vi "Test Get VIs.vi"(8 "Error In":errorcluster) -> ()   [LabVIEW 2018]
uses:
  <vilib>/Utility/traverseref.llb/TRef TravTarget.ctl
  <vilib>/Utility/traverseref.llb/VI Scripting - Traverse.lvlib
panel:
  out "Wires and connected ClassNames in for loop.":string[][](array[string])
  out "Objects[] in for loop":string[](array[string])
  out "All Objects[]":string[](array[string])
  in  "vi path":path=path "C:/Users/lubo/Documents/LabView/LabVIEW-Universal-Transcriptor/Test/Examples For Parsing/Example Test 1.vi"
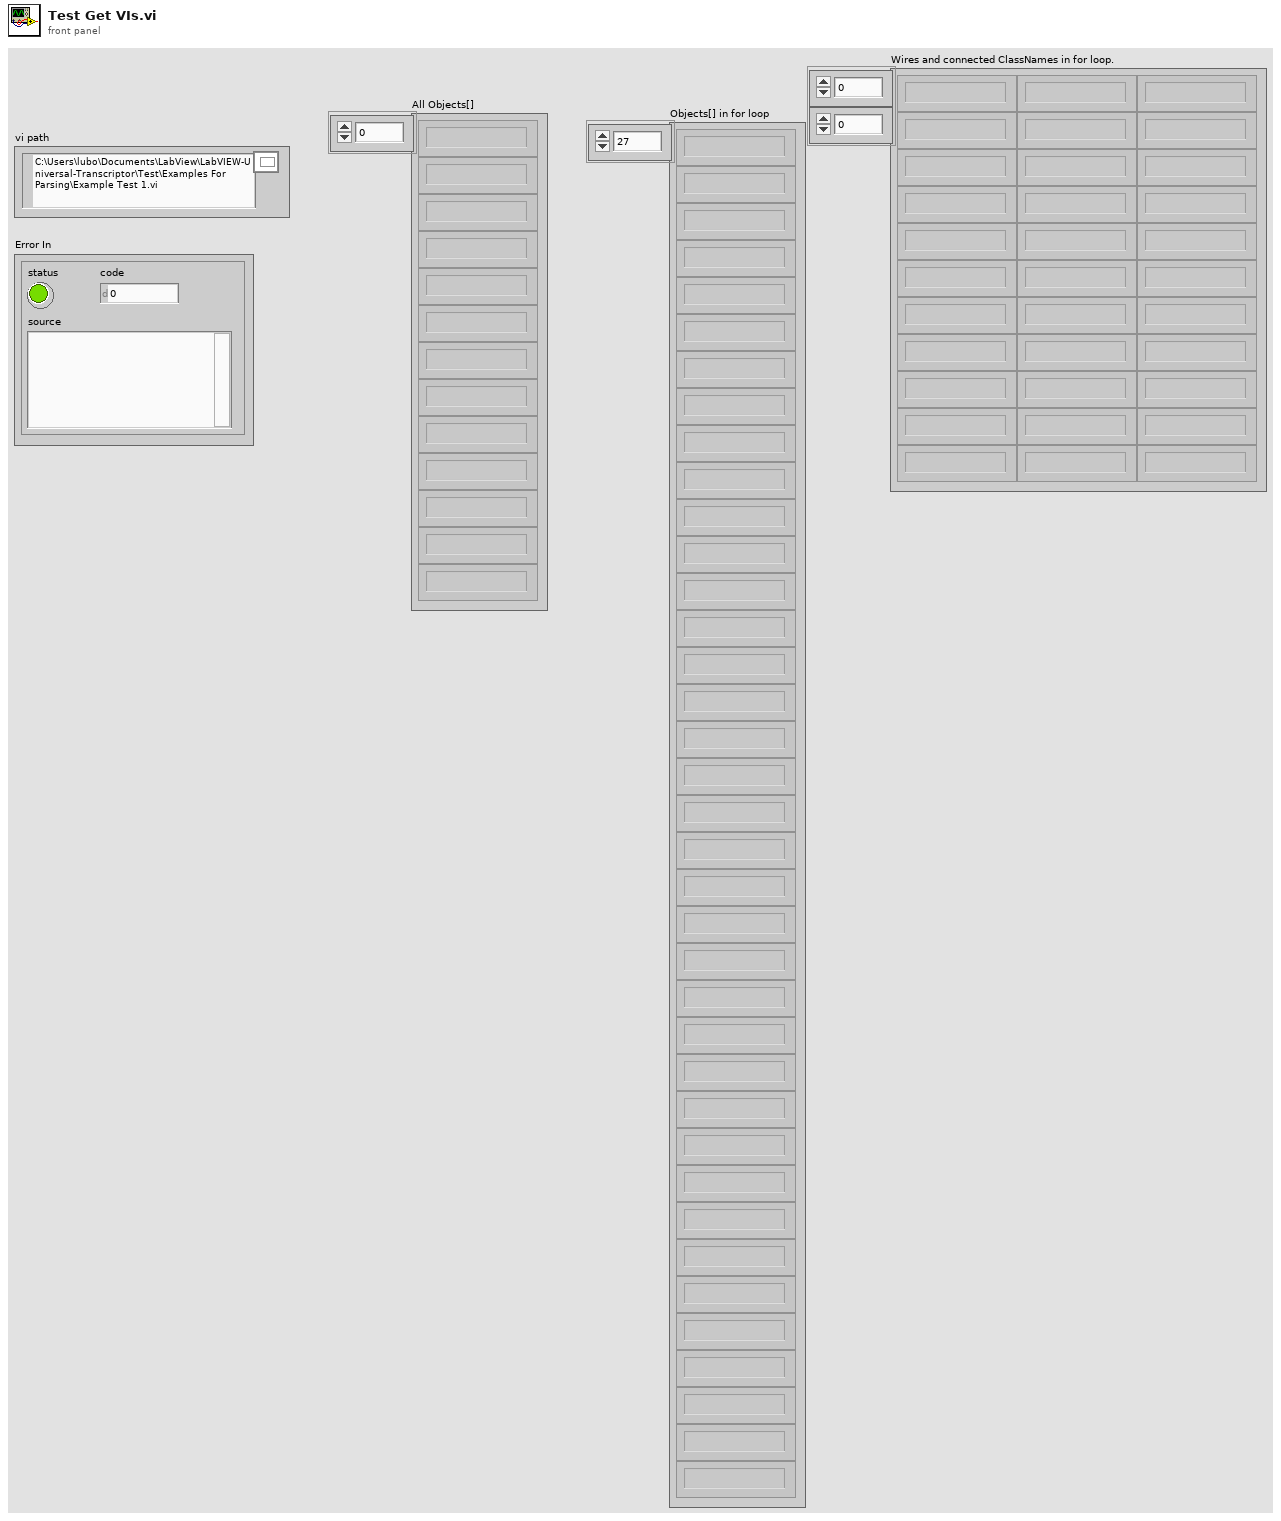
[diagram p1: front panel]
types:
  T1 = typedef "TRef TravTarget.ctl" = enum16{"FP", "BD", "Other"}
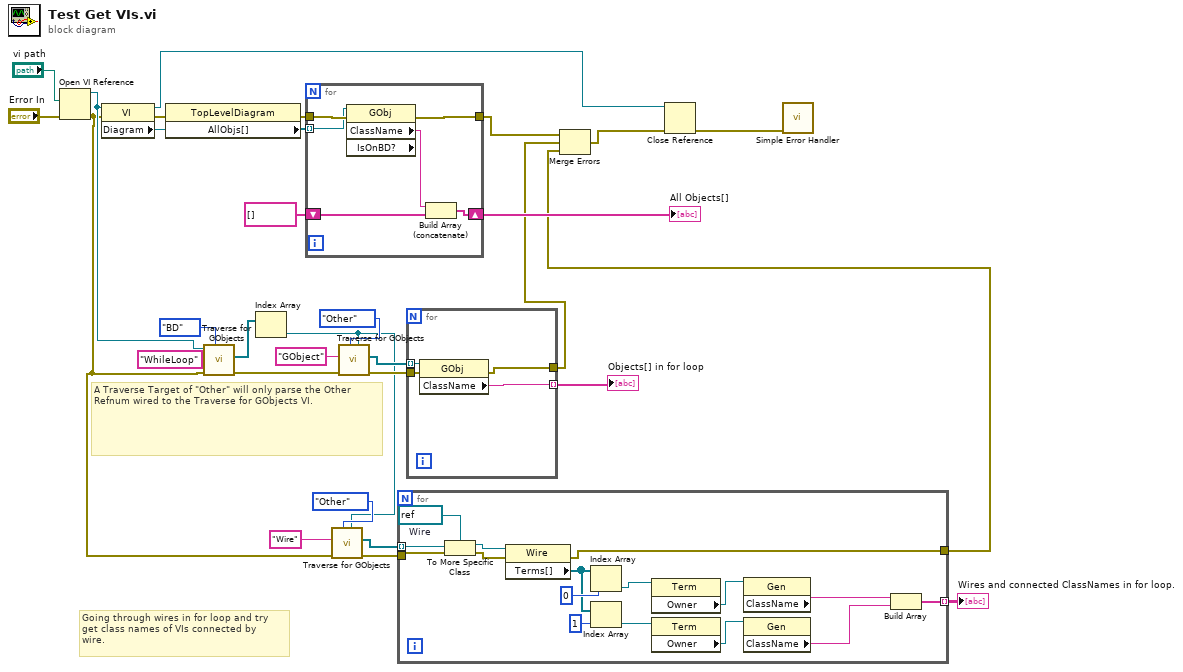
[diagram p0: block diagram]
diagram:
  # "Going through wires in for loop and try\nget class names of VIs connected by\nwire."
  # "A Traverse Target of \"Other\" will only parse the Other Refnum wired to the Traverse for GObjects VI."
  n1 = Open VI Reference(vi path="vi path", error in (no error)="Error In") -> (vi reference=w17:refnum<vi>, error out=w4:errorcluster)  [unwired: 4 in]
  n2 = property class="VI"(reference=w17, error in=w4) -> (reference out=w29:refnum<vi>, error out=w27:errorcluster, "Diagram"=w28:refnum<vi>)
  n3 = property class="TopLevelDiagram"(reference=w28, error in=w27) -> (error out=w25:errorcluster, "AllObjs[]"=w24:refnum<vi>[])  [unwired: 1 out]
  n4 = call <vilib>:"Traverse for GObjects.vi"("Traverse Target"=TRef_TravTarget."BD", "error in (no error)"=w4, "Class Name"="WhileLoop", "VI Refnum"=w17) -> ("error out"=w20:errorcluster, "References"=w21:refnum<vi>[])  [unwired: 4 in, 2 out]
  n5 = Index Array(array=w21) -> (element=w5:refnum<vi>)  [unwired: 1 in]
  n6 = for {
    tunnel: w25 -> [w37]
    tunnel: w24 -> [w36] mode=indexing
    shift-right: [w33] -> w23
    shift-left: string[] [] -> [w34]
    tunnel: [w32] -> w12
    n7 = property class="GObj" props=["ClassName", "IsOnBD?"](reference=w36, error in=w37) -> (error out=w32:errorcluster, "ClassName"=w35:string)  [unwired: 2 out]
    n8 = Build Array (concatenate)(w35, w34) -> (w33:string[])
  }
  "All Objects[]" <- w23
  n9 = call <vilib>:"Traverse for GObjects.vi"("Other Refnum"=w5, "Traverse Target"=TRef_TravTarget."Other", "error in (no error)"=w4, "Class Name"="Wire") -> ("error out"=w8:errorcluster, "References"=w9:refnum<vi>[])  [unwired: 4 in, 2 out]
  n10 = call <vilib>:"Traverse for GObjects.vi"("Other Refnum"=w5, "Traverse Target"=TRef_TravTarget."Other", "error in (no error)"=w20, "Class Name"="GObject") -> ("error out"=w15:errorcluster, "References"=w14:refnum<vi>[])  [unwired: 4 in, 2 out]
  n11 = for {
    tunnel: w8 -> [w51]
    tunnel: w9 -> [w52] mode=indexing
    tunnel: [w53] -> w3
    tunnel: [w43] -> w2 mode=indexing
    w50 = refnum<vi> refnum  # Wire
    n12 = To More Specific Class(target class=w50, reference=w52, error in=w51) -> (specific class reference=w49:refnum<vi>, error out=w48:errorcluster)
    n13 = property class="Wire"(reference=w49, error in=w48) -> (error out=w53:errorcluster, "Terms[]"=w38:refnum<vi>[])  [unwired: 1 out]
    n14 = Index Array(array=w38, index=0) -> (element=w45:refnum<vi>)
    n15 = Index Array(array=w38, index=1) -> (element=w44:refnum<vi>)
    n16 = property class="Term"(reference=w45) -> ("Owner"=w42:refnum<vi>)  [unwired: 1 in, 2 out]
    n17 = property class="Term"(reference=w44) -> ("Owner"=w41:refnum<vi>)  [unwired: 1 in, 2 out]
    n18 = property class="Gen"(reference=w42) -> ("ClassName"=w39:string)  [unwired: 1 in, 2 out]
    n19 = property class="Gen"(reference=w41) -> ("ClassName"=w40:string)  [unwired: 1 in, 2 out]
    n20 = Build Array(w39, w40) -> (w43:string[])
  }
  "Wires and connected ClassNames in for loop." <- w2
  n21 = for {
    tunnel: w15 -> [w57]
    tunnel: w14 -> [w56] mode=indexing
    tunnel: [w55] -> w13 mode=indexing
    tunnel: [w54] -> w11
    n22 = property class="GObj"(reference=w56, error in=w57) -> (error out=w54:errorcluster, "ClassName"=w55:string)  [unwired: 1 out]
  }
  "Objects[] in for loop" <- w13
  n23 = Merge Errors(w12, w11, w3) -> (w10:errorcluster)
  n24 = Close Reference(reference=w29, error in (no error)=w10) -> (error out=w30:errorcluster)
  n25 = call <vilib>:"Simple Error Handler.vi"("error in (no error)"=w30) -> ()  [unwired: 4 in, 5 out]
